vi "Init.vi"(8 "error in (no error)":errorcluster, 9 "Maximum length of Frames buffer":i32=10000, 10 "COM port":refnum<visa-resource-name>) -> (0 "error out":errorcluster, 3 "uCAN out":refnum<class "uCAN.lvclass">)   [LabVIEW 2021, in "uCanDriver.lvlib" / "uCAN.lvclass"]
doc: "Initialise uCAN device on given COM port"
uses:
  uCAN.lvclass
  typedefs/frame.ctl
  uCAN.lvclass/uCAN.ctl
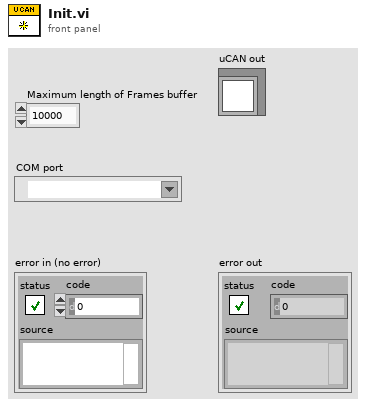
[diagram p1: front panel]
types:
  T1 = typedef "uCanDriver.lvlib/uCAN.lvclass/frame.ctl" = cluster{"Extended":bool, "ID":u32, "Data":u8[], "DLC":u8}
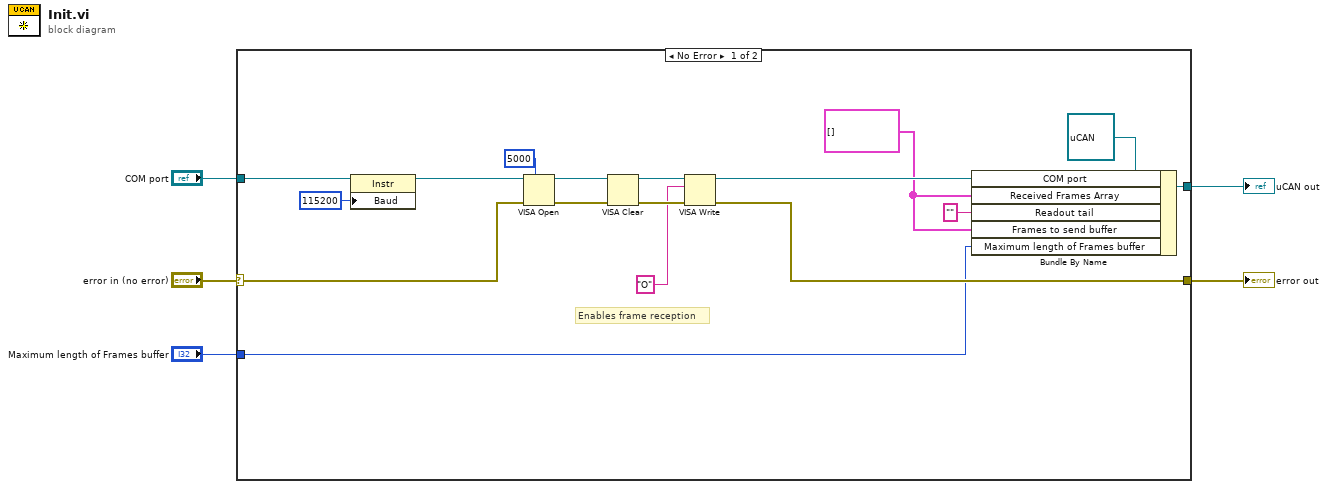
[diagram p0: block diagram]
diagram:
  n1 = case shown="No Error" "error in (no error)" {
    selector: "error in (no error)" -> [w14 w23]
    tunnel: [w13 w23] -> w4
    tunnel: [w21 _] -> w3
    tunnel: "COM port" -> [w11 _]
    tunnel: "Maximum length of Frames buffer" -> [w6 _]
    frame No Error {
      w7 = T1[] [] ("Received Frames Array")
      # "Enables frame reception"
      n2 = property class="Instr"(reference=w11, "Baud"=u32 115200 ("Serial Settings:Baud Rate")) -> (reference out=w10:refnum<visa-resource-name>)  [unwired: 1 in, 1 out]
      n3 = VISA Open(timeout (0)=u32 5000 ("VISA Open timeout (0)"), error in (no error)=w14, VISA resource name=w10) -> (VISA resource name=w18:refnum<visa-resource-name>, error out=w19:errorcluster)  [unwired: 2 in]
      n4 = VISA Clear(VISA resource name=w18, error in (no error)=w19) -> (VISA resource name out=w17:refnum<visa-resource-name>, error out=w16:errorcluster)
      n5 = VISA Write(VISA resource name=w17, write buffer="O", error in (no error)=w16) -> (VISA resource name out=w12:refnum<visa-resource-name>, error out=w13:errorcluster)  [unwired: 1 out]
      n6 = Bundle By Name(cluster=refnum<class "uCAN.lvclass"> refnum ("uCAN out"), "COM port"=w12, "Received Frames Array"=w7, "Readout tail"="", "Frames to send buffer"=w7, "Maximum length of Frames buffer"=w6) -> (w21:refnum<class "uCAN.lvclass">)
    }
    frame Error {
    }
  }
  "error out" <- w4
  "uCAN out" <- w3
